vi "Combine File Lists.vi"(8 "error in":errorcluster, 11 "Peer Review in":refnum<class "Peer Review.lvclass">) -> (0 "error out":errorcluster, 3 "Peer Review out":refnum<class "Peer Review.lvclass">)   [LabVIEW 2020, in "Peer Review.lvclass"]
uses:
  Peer Review.lvclass
  TypeDefs/File Info.ctl
  TypeDefs/File State.ctl
  TypeDefs/VI Type.ctl
  Peer Review.lvclass/Peer Review.ctl
  bc492ac1-b37c-4842-bcf3-d3358cf64c6e.vi
  <vilib>/security/Message Digest/API/Instances/File/SHA-256 File Checksum.vi
  <vilib>/security/Message Digest/API/NI_Message Digest API.lvlib
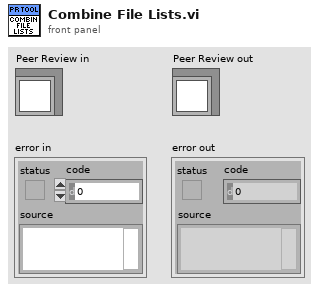
[diagram p1: front panel]
types:
  T1 = typedef "Peer Review.lvclass/File Info.ctl" = cluster{"File ID":i32, "Commit ID":i32, "Reviewed Hash":string, "Relative Path":string, "File Path":path, "File Checksum":string, "State":T2, "FP Changes":i32, "BD Changes":i32, "FP Bounds Error":dbl, "BD Bounds Error":dbl, "Lines Added":i32, "Lines Removed":i32, "Analysis Passes":i32, "Analysis Fails":i32, "Attribute Changes":i32, "Reentrancy State":string, "Cyclomatic Complexity":i32, "Node Count":i32, "Revision Number":u32, "LabVIEW Version":string, "Description":string, "Master Path":path, "Master Checksum":string, "VI Type":T3, "LabVIEW File":bool, "Review Complete":bool, "File Ref":refnum<vi>}
  T2 = typedef "Peer Review.lvclass/File State.ctl" = enum16{"Interrogation Needed", "Modified", "Deleted", "Added", "Matches Previous", "No Changes", "Moved"}
  T3 = typedef "Peer Review.lvclass/VI Type.ctl" = enum32{"invalid VI type", "Standard VI", "Control VI", "Global VI", "Polymorphic VI", "Configuration VI", "SubSystem", "Facade VI", "Method VI", "Statechart Diagram VI"}
  T4 = typedef "Peer Review.lvclass/Commit Info.ctl" = cluster{"Commit ID":i32, "Hash":string, "Merge Commit?":bool, "Merge Hash":string, "Author":string, "Time Stamp":timestamp, "Description":string, "File Count":i32, "File List":string[]}
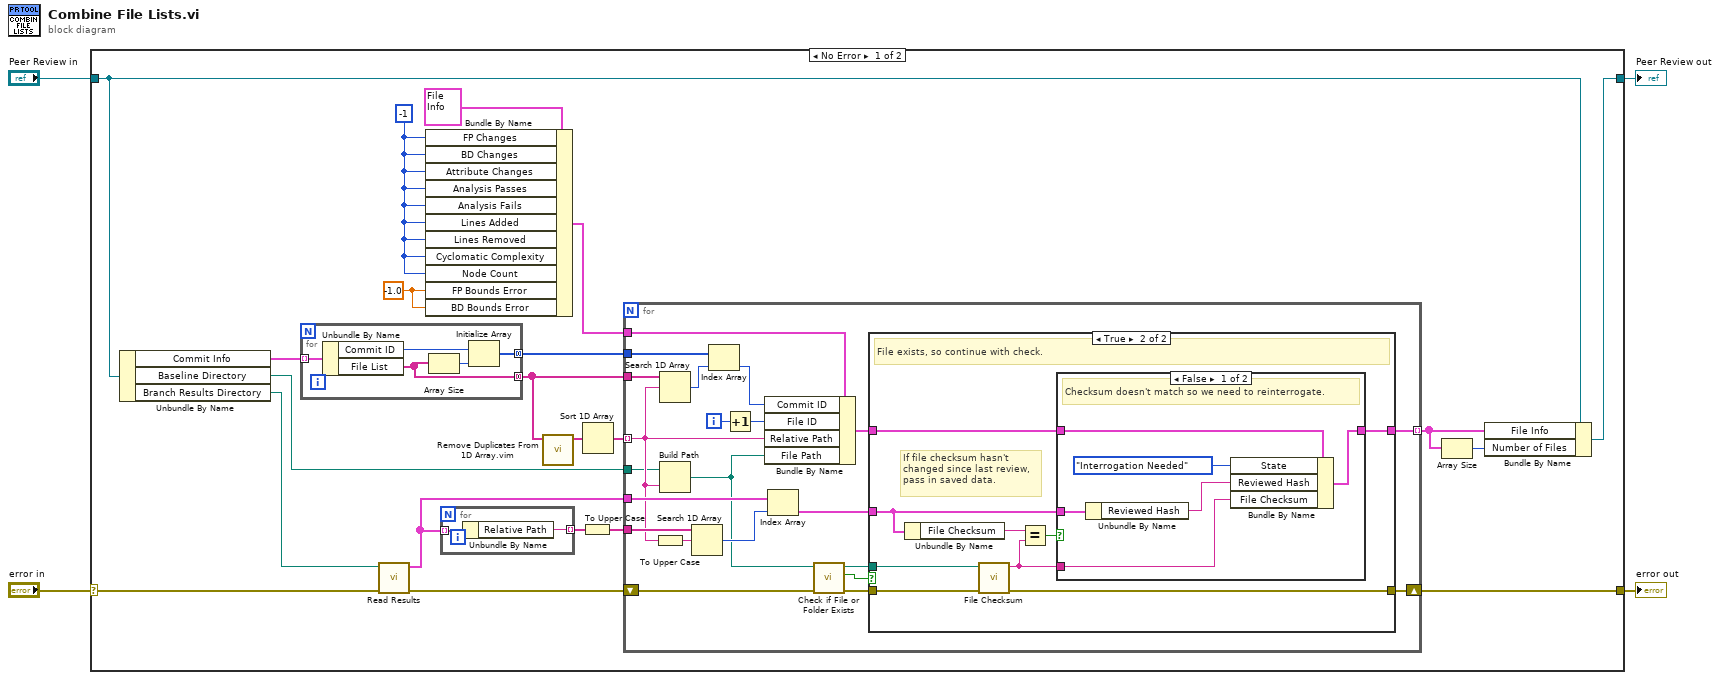
[diagram p0: block diagram]
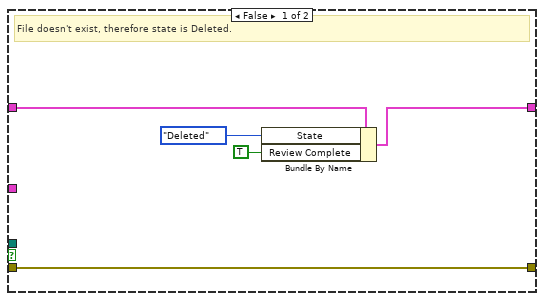
[diagram p2: hidden frame]
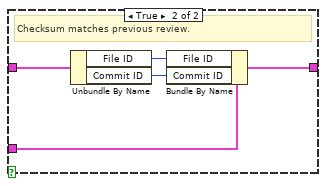
[diagram p3: hidden frame]
diagram:
  n1 = case shown="No Error" "error in" {
    selector: "error in" -> [w19 w80]
    tunnel: "Peer Review in" -> [w25 w81]
    tunnel: [w7 w81] -> w3
    tunnel: [w13 w80] -> w1
    frame No Error {
      w5 = -1.0 ("FP Bounds Error")
      w6 = -1 ("FP Changes")
      n2 = Unbundle By Name(w25) -> ("Commit Info"=w20:T4[], "Baseline Directory"=w14:path, "Branch Results Directory"=w17:path)
      n3 = for {
        tunnel: w20 -> [w79] mode=indexing
        tunnel: [w76] -> w22 mode=concatenating
        tunnel: [w77] -> w21 mode=concatenating
        n4 = Unbundle By Name(w79) -> ("Commit ID"=w75:i32, "File List"=w76:string[])
        n5 = Array Size(array=w76) -> (size(s)=w78:i32)
        n6 = Initialize Array(w75, w78) -> (w77:i32[])
      }
      n7 = call "Read Results.vi"("error in"=w19, "Results Directory"=w17) -> ("error out"=w18:errorcluster, "Results"=w16:T1[])  [unwired: 8 in]
      n8 = Bundle By Name(cluster=T1 {"File ID"=0, "Commit ID"=0, "Reviewed Hash"="", "Relative Path"="", "File Path"=path "", "File Checksum"="", "State"=enum."Interrogation Needed", "FP Changes"=0, "BD Changes"=0, "FP Bounds Error"=0.0, "BD Bounds Error"=0.0, "Lines Added"=0, "Lines Removed"=0, "Analysis Passes"=0, "Analysis Fails"=0, "Attribute Changes"=0, "Reentrancy State"="", "Cyclomatic Complexity"=0, "Node Count"=0, "Revision Number"=0, "LabVIEW Version"="", "Description"="", "Master Path"=path "", "Master Checksum"="", "VI Type"=enum."invalid VI type", "LabVIEW File"=FALSE, "Review Complete"=FALSE, "File Ref"=refnum} ("Compare Info"), "FP Changes"=w6, "BD Changes"=w6, "Attribute Changes"=w6, "Analysis Passes"=w6, "Analysis Fails"=w6, "Lines Added"=w6, "Lines Removed"=w6, "Cyclomatic Complexity"=w6, "Node Count"=w6, "FP Bounds Error"=w5, "BD Bounds Error"=w5) -> (w11:T1)
      n9 = for {
        tunnel: w16 -> [w27] mode=indexing
        tunnel: [w26] -> w15 mode=indexing
        n10 = Unbundle By Name(w27) -> ("Relative Path"=w26:string)
      }
      n11 = call "Remove Duplicates From 1D Array.vim"("array"=w22) -> ("array with duplicates removed"=w23:string[])  [unwired: 10 in]
      n12 = To Upper Case(1:w15) -> (0:w10:string[])
      n13 = Sort 1D Array(array=w23) -> (sorted array=w24:string[])
      n14 = for {
        tunnel: w24 -> [w32] mode=indexing
        tunnel: [w35] -> w9 mode=indexing
        tunnel: w22 -> [w48]
        tunnel: w21 -> [w47]
        shift-right: [w37] -> w13
        shift-left: w18 -> [w40]
        tunnel: w16 -> [w39]
        tunnel: w10 -> [w38]
        tunnel: w14 -> [w30]
        tunnel: w11 -> [w29]
        i -> [w49]
        n15 = To Upper Case(1:w32) -> (0:w28:string)
        n16 = Search 1D Array(1D array=w48, element=w32) -> (index of element=w46:i32)  [unwired: 1 in]
        n17 = Build Path(base path=w30, name or relative path=w32) -> (appended path=w33:path)
        n18 = Search 1D Array(1D array=w38, element=w28) -> (index of element=w42:i32)  [unwired: 1 in]
        n19 = Index Array(array=w47, index=w46) -> (element=w34:i32)
        n20 = Increment(x=w49) -> (x+1=w31:i32)
        n21 = Bundle By Name(cluster=w29, "Commit ID"=w34, "File ID"=w31, "Relative Path"=w32, "File Path"=w33) -> (w36:T1)
        n22 = Index Array(array=w39, index=w42) -> (element=w41:T1)
        n23 = call <vilib>:"Check if File or Folder Exists.vi"("error in (no error)"=w40, "path"=w33) -> ("error out"=w45:errorcluster, "file or folder exists?"=w43:bool, "dup path"=w44:path)  [unwired: 7 in]
        n24 = case shown="True" w43 {
          tunnel: [w54 w55] -> w37
          tunnel: w45 -> [w54 w56]
          tunnel: w44 -> [_ w58]
          tunnel: w41 -> [_ w61]
          tunnel: w36 -> [w51 w62]
          tunnel: [w52 w57] -> w35
          frame False {
            # "File doesn't exist, therefore state is Deleted."
            n25 = Bundle By Name(cluster=w51, "State"=File_State."Deleted", "Review Complete"=TRUE) -> (w52:T1)
          }
          frame True {
            # "If file checksum hasn't\nchanged since last review,\npass in saved data."
            # "File exists, so continue with check."
            n26 = Unbundle By Name(w61) -> ("File Checksum"=w63:string)
            n27 = call-poly <vilib>:"File Checksum.vi"("error in"=w56, "path"=w58) -> ("error out"=w55:errorcluster, "digest"=w60:string)  [unwired: 8 in]
            n28 = Equal?(x=w63, y=w60) -> (x = y?=w59:bool)
            n29 = case shown="False" w59 {
              tunnel: w62 -> [w67 w73]
              tunnel: w61 -> [w65 w70]
              tunnel: [w66 w74] -> w57
              tunnel: w60 -> [w68 _]
              frame False {
                # "Checksum doesn't match so we need to reinterrogate."
                n30 = Unbundle By Name(w65) -> ("Reviewed Hash"=w64:string)
                n31 = Bundle By Name(cluster=w67, "State"=File_State."Interrogation Needed", "Reviewed Hash"=w64, "File Checksum"=w68) -> (w66:T1)
              }
              frame True {
                # "Checksum matches previous review."
                n32 = Unbundle By Name(w73) -> ("File ID"=w72:i32, "Commit ID"=w71:i32)
                n33 = Bundle By Name(cluster=w70, "File ID"=w72, "Commit ID"=w71) -> (w74:T1)
              }
            }
          }
        }
      }
      n34 = Array Size(array=w9) -> (size(s)=w8:i32)
      n35 = Bundle By Name(cluster=w25, "File Info"=w9, "Number of Files"=w8) -> (w7:refnum<class "Peer Review.lvclass">)
    }
    frame Error {
    }
  }
  "error out" <- w1
  "Peer Review out" <- w3
